vi "Output (Character Codes).vi"(8 "error in (no error)":errorcluster, 9 "position":cluster{"row":i8, "column":i8}, 10 "character codes":u8[](array[numeric]), 11 "LCD in":refnum<class "Character LCD.lvclass">) -> (0 "error out":errorcluster, 1 "current cursor position":cluster{"row":i8, "column":i8}, 3 "LCD out":refnum<class "Character LCD.lvclass">)   [LabVIEW 2017, in "HD44780 Host.lvlib"]
uses:
  HD44780 Host.lvlib
  Internal/LCD Class/Character LCD.lvclass
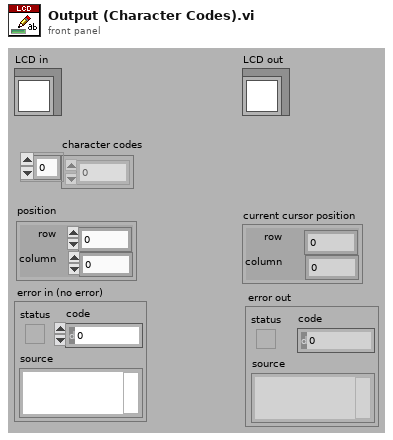
[diagram p1: front panel]
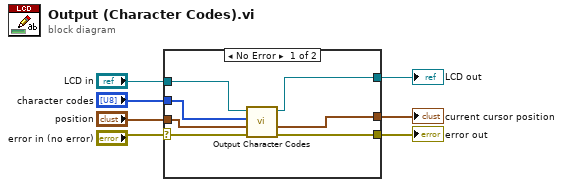
[diagram p0: block diagram]
diagram:
  n1 = case shown="No Error" "error in (no error)" {
    selector: "error in (no error)" -> [w12 w17]
    tunnel: [w10 w17] -> w4
    tunnel: "character codes" -> [w14 _]
    tunnel: "position" -> [w13 w15]
    tunnel: "LCD in" -> [w11 w16]
    tunnel: [w9 w16] -> w2
    tunnel: [w8 w15] -> w1
    frame No Error {
      n2 = call-dynamic "Output Character Codes.vi"("error in (no error)"=w12, "position"=w13, "character codes"=w14, "Character LCD in"=w11) -> ("error out"=w10:errorcluster, "current cursor position"=w8:cluster{"row":i8, "column":i8}, "Character LCD out"=w9:refnum<class "Character LCD.lvclass">)  [unwired: 5 in]
    }
    frame Error {
    }
  }
  "error out" <- w4
  "LCD out" <- w2
  "current cursor position" <- w1
